vi "Run.vi"(0 "reg in":refnum<class "bronkhorst_reg.lvclass">, 1 "XB24 (F)":bool, 5 "SP":dbl caption="setpoint" step=0.01 format="%.2f", 7 "PV":dbl step=0.01 format="%.2f", 9 "PV_State":T5, 11 "error in (no error)":errorcluster, 12 "Y_in":dbl step=0.01 format="%.2f", 13 "Y_State":T5) -> (4 "reg out":refnum<class "bronkhorst_reg.lvclass">, 6 "Y_out":dbl format="%.2f", 8 "T":u32, 10 "End":bool, 15 "error out":errorcluster)   [LabVIEW 2019, in "bronkhorst_reg.lvclass"]
uses:
  bronkhorst_reg.lvclass
  Inputs/Ctl/Parameter State short.ctl
  ctl/Y_Lim_State.ctl
  ctl/ZY_control_short.ctl
  ctl/Z_State.ctl
  ctl/Y_state.ctl
  bronkhorst_reg.lvclass/bronkhorst_reg.ctl
  ctl/control param simple.ctl
  PID/PID Output Rate Limiter Ext.vi
  PID/PID Timing Estimation Ext.vi
  control.lvlib
  Inputs/Inputs.lvlib
panel:
  out "ZY_control":T1={"Start"=FALSE, "Z_HSw"=0, "Z_HSetState"=enum."on", "Y_HSw"=0, "Y_HSetState"=enum."hand", "SP"=0.0, "Y_H"=0.0, "Reset_ALR"=FALSE} {"Y_H" step=1.0; "SP" step=0.01 format="%.2f"}
  out "SpLim_State":T4=enum."increase"
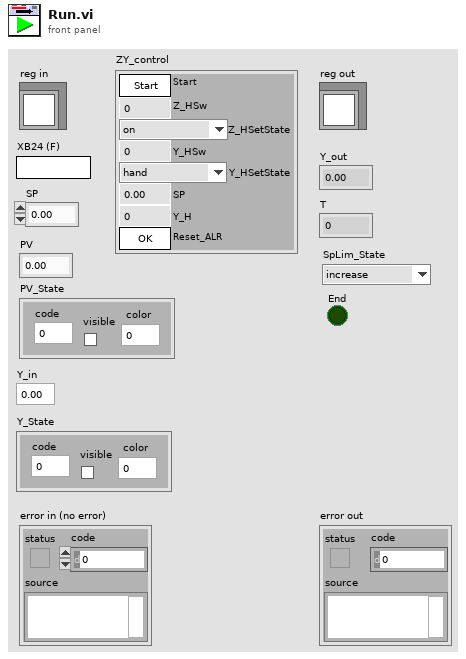
[diagram p1: front panel]
types:
  T1 = typedef "control.lvlib/ZY_control_short.ctl" = cluster{"Start":bool, "Z_HSw":u32, "Z_HSetState":T2, "Y_HSw":u32, "Y_HSetState":T3, "SP":dbl, "Y_H":dbl, "Reset_ALR":bool}
  T2 = typedef "control.lvlib/Z_State.ctl" = enum8{"initialization", "alarm", "disabled", "not ready", "stop ready", "reserv", "switched off", "reserv2", "switched on", "check", "on min", "decrease out", "on", "increase out", "on max"}
  T3 = typedef "control.lvlib/Y_state.ctl" = enum8{"initialize", "alarm", "min", "stop", "hand", "auto", "max"}
  T4 = typedef "control.lvlib/Y_Lim_State.ctl" = enum8{"initialization", "alarm", "stop", "decrease", "increase"}
  T5 = typedef "Inputs.lvlib/Parameter State short.ctl" = cluster{"code":i32, "visible":bool, "color":u32}
  T6 = typedef "control.lvlib/control param simple.ctl" = cluster{"output high":dbl, "alr value":dbl, "output low":dbl, "output time (t)":dbl}
  T7 = cluster{"Y_HSw":u32, "Y_HSetState":T3, "Y_ASetState":T3, "Y_DSetState":T3}
  T8 = typedef "control.lvlib/control param.ctl" = cluster{"proportional gain (Kc)":dbl, "integral time (Ti, s)":dbl, "derivative time (Td, s)":dbl, "output high":dbl, "output high start":dbl, "output high stop":dbl, "alr value":dbl, "output low":dbl, "output rate (EGU/s)":dbl, "setpoint max":dbl, "setpoint rate (EGU/min)":dbl, "stop rate (EGU/min)":dbl}
  T9 = typedef "control.lvlib/Y_source.ctl" = enum8{"initialize", "local disabled", "local hand", "hand", "auto", "dist"}
  T10 = enum8{"alarm", "min", "stop", "hand", "auto", "max"}
  T11 = typedef "control.lvlib/Y_Lim_ext_defs.ctl" = cluster{"reinitialize":bool, "SpLim_State":T4, "output":dbl, "Tick":u32, "output rate":dbl, "Y_Set":dbl, "Y_preSet":dbl}
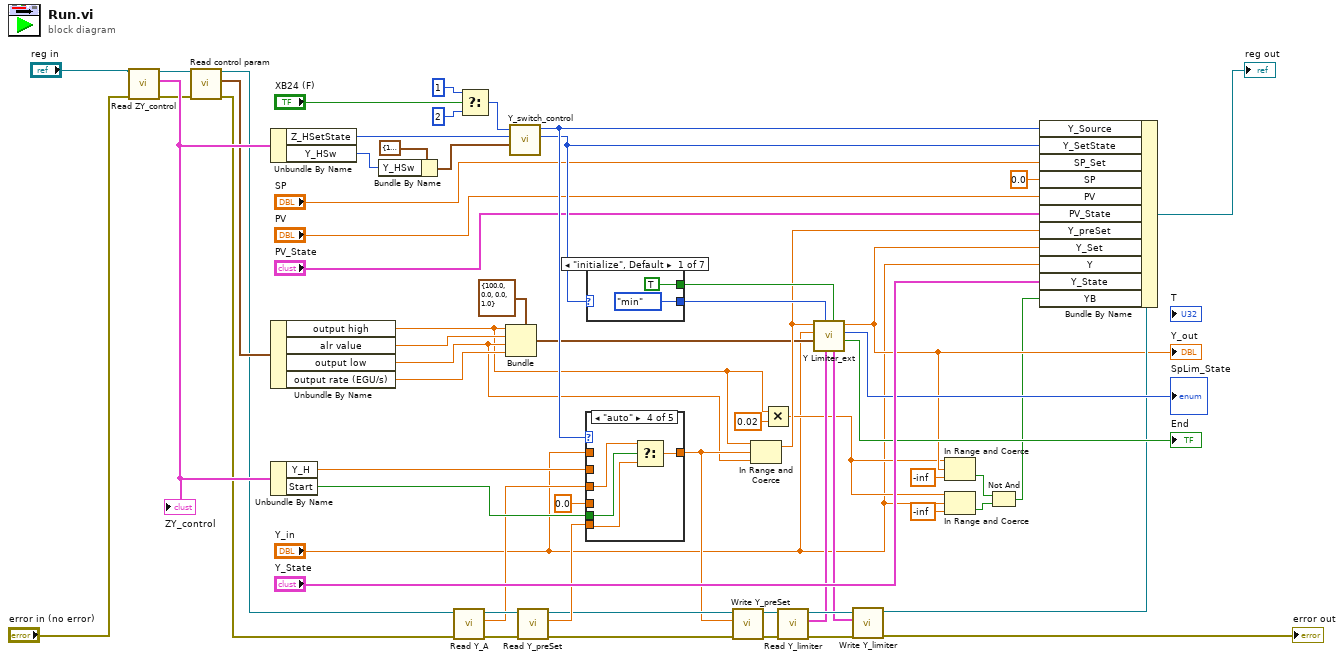
[diagram p0: block diagram]
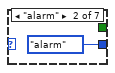
[diagram p2: hidden frame]
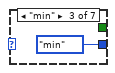
[diagram p3: hidden frame]
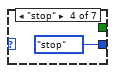
[diagram p4: hidden frame]
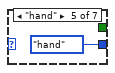
[diagram p5: hidden frame]
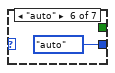
[diagram p6: hidden frame]
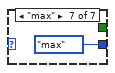
[diagram p7: hidden frame]
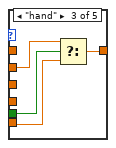
[diagram p10: hidden frame]
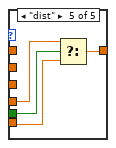
[diagram p11: hidden frame]
diagram:
  n1 = call "Read ZY_control.vi"("error in (no error)"="error in (no error)", "reg in"="reg in") -> ("error out"=w22:errorcluster, "ZY_control"=w26:T1, "reg out"=w23:refnum<class "bronkhorst_reg.lvclass">)  [unwired: 7 in]
  "ZY_control" <- w26
  n2 = call "Read control param.vi"("error in (no error)"=w22, "reg in"=w23) -> ("error out"=w14:errorcluster, "control param"=w21:T8, "reg out"=w15:refnum<class "bronkhorst_reg.lvclass">)  [unwired: 7 in]
  n3 = Unbundle By Name(w26) -> ("Z_HSetState"=w30:T2, "Y_HSw"=w33:u32)
  n4 = Unbundle By Name(w21) -> ("output high"=w9:dbl, "alr value"=w18:dbl, "output low"=w16:dbl, "output rate (EGU/s)"=w17:dbl)
  n5 = Unbundle By Name(w26) -> ("Y_H"=w24:dbl, "Start"=w25:bool)
  n6 = Bundle By Name(cluster=T7 {"Y_HSw"=1, "Y_HSetState"=enum."hand", "Y_ASetState"=enum."hand", "Y_DSetState"=enum."auto"} ("Y_Set"), "Y_HSw"=w33) -> (w29:T7)
  n7 = call "Read Y_A.vi"("error in (no error)"=w14, "reg in"=w15) -> ("error out"=w12:errorcluster, "Y_A"=w11:dbl, "reg out"=w13:refnum<class "bronkhorst_reg.lvclass">)  [unwired: 7 in]
  n8 = Select(t=u32 1, s="XB24 (F)", f=u32 2 ("Y_HSw")) -> (s? t:f=w60:u32)
  n9 = Bundle(cluster=T6 {"output high"=100.0, "alr value"=0.0, "output low"=0.0, "output time (t)"=1.0} ("control param"), "output high"=w9, "alr value"=w18, "output low"=w16, "output time (t)"=w17) -> (w19:T6)
  n10 = call "Y_switch_control.vi"("Y"=w29, "Z_State"=w30, "Y_LSw (2-auto)"=w60) -> ("Y_SetState"=w57:T3, "Y_Source"=w58:T9)  [unwired: 7 in]
  n11 = call "Read Y_preSet.vi"("error in (no error)"=w12, "reg in"=w13) -> ("error out"=w41:errorcluster, "Y_preSet"=w46:dbl, "reg out"=w45:refnum<class "bronkhorst_reg.lvclass">)  [unwired: 7 in]
  n12 = case shown="\"auto\"" w58 {
    tunnel: w24 -> [_ _ w65 _ _]
    tunnel: "Y_in" -> [w63 w64 _ _ _]
    tunnel: 0.0 ("Y_A") -> [_ _ _ _ w75]
    tunnel: [w63 w64 w68 w72 w76] -> w44
    tunnel: w11 -> [_ _ _ w69 _]
    tunnel: w46 -> [_ _ w67 w71 w74]
    tunnel: w25 -> [_ _ w66 w70 w73]
    frame "local disabled", Default {
    }
    frame "local hand" {
    }
    frame "hand" {
      n13 = Select(t=w65, s=w66, f=w67) -> (s? t:f=w68:dbl)
    }
    frame "auto" {
      n14 = Select(t=w69, s=w70, f=w71) -> (s? t:f=w72:dbl)
    }
    frame "dist" {
      n15 = Select(t=w75, s=w73, f=w74) -> (s? t:f=w76:dbl)
    }
  }
  n16 = case shown="\"initialize\", Default" w57 {
    tunnel: [T10."min" ("X1(SetState)") T10."alarm" ("X1(SetState)") T10."min" ("X1(SetState)") T10."stop" ("X1(SetState)") T10."hand" ("X1(SetState)") T10."auto" ("X1(SetState)") T10."max" ("X1(SetState)")] -> w51
    tunnel: [TRUE _ _ _ _ _ _] -> w52
    frame "initialize", Default {
    }
    frame "alarm" {
    }
    frame "min" {
    }
    frame "stop" {
    }
    frame "hand" {
    }
    frame "auto" {
    }
    frame "max" {
    }
  }
  n17 = call "Write Y_preSet.vi"("error in (no error)"=w41, "Y_preSet"=w44, "reg in"=w45) -> ("error out"=w42:errorcluster, "reg out"=w43:refnum<class "bronkhorst_reg.lvclass">)  [unwired: 7 in]
  n18 = In Range and Coerce(upper limit=w9, x=w44, lower limit=w16) -> (coerced(x)=w47:dbl)  [unwired: 1 out]
  n19 = Multiply(x=w9, y=0.02) -> (x*y=w5:dbl)
  n20 = call "Read Y_limiter.vi"("error in (no error)"=w42, "reg in"=w43) -> ("error out"=w38:errorcluster, "Y_limiter"=w39:T11, "reg out"=w40:refnum<class "bronkhorst_reg.lvclass">)  [unwired: 7 in]
  n21 = call "Y Limiter_ext.vi"("reinitialize? (F)"=w52, "Y_limiter_old"=w39, "X1(SetState)"=w51, "Y param"=w19, "Y (NaN)"="Y_in", "Y_Set"=w47) -> ("End"=→"End":bool, "SpLim_State"=→"SpLim_State":T4, "output"=w7:dbl, "Y_limiter"=w37:T11)  [unwired: 2 in]
  "Y_out" <- w7
  n22 = call "Write Y_limiter.vi"("error in (no error)"=w38, "Y_limiter"=w37, "reg in"=w40) -> ("error out"=→"error out":errorcluster, "reg out"=w36:refnum<class "bronkhorst_reg.lvclass">)  [unwired: 7 in]
  n23 = In Range and Coerce(upper limit=w5, x=w7, lower limit=-inf) -> (In Range?=w3:bool)  [unwired: 1 out]
  n24 = In Range and Coerce(upper limit=w5, x="Y_in", lower limit=-inf) -> (In Range?=w2:bool)  [unwired: 1 out]
  n25 = Not And(1:w2, 2:w3) -> (0:w1:bool)
  n26 = Bundle By Name(cluster=w36, "Y_Source"=w58, "Y_SetState"=w57, "SP_Set"="SP", "SP"=0.0, "PV"="PV", "PV_State"="PV_State", "Y_preSet"=w47, "Y_Set"=w7, "Y"="Y_in", "Y_State"="Y_State", "YB"=w1) -> (→"reg out":refnum<class "bronkhorst_reg.lvclass">)
